vi "Streamlined FPGA--130415.vi"() -> ()   [LabVIEW 2009]
uses:
  Instance           2 24Saved   Streamlined FPGA .vi
  <vilib>/eio/EIONode/EIONode.xnode
  Instance           3 24Saved   Streamlined FPGA .vi
  Instance           4 24Saved   Streamlined FPGA .vi
  Instance           5 24Saved   Streamlined FPGA .vi
  <vilib>/rvi/eio/nirviEIOImplementation/nirviEIOImplementation.xnode
  <vilib>/rvi/eio/common/nirviEmuClasses.ctl
  <vilib>/rvi/eio/common/nirviEmuTemplateMethod_noerrors.vi
  <vilib>/rvi/DataTransferAndStorage/Container/XNode/niFpgaContainer.xnode
  <vilib>/rvi/DataTransferAndStorage/Container/Common/niFpgaTransferTypeControl.ctl
  <vilib>/rvi/DataTransferAndStorage/Container/Common/niFpgaContainerMethod.ctl
  <vilib>/rvi/interface/RandomDataEmulation/nirviRandomDataFPGAFIFO.vi
  <vilib>/rvi/interface/RandomDataEmulation/niFpgaRandomDataHandleErrors.vi
panel:
  in  "window size":i32
  in  "smooth":bool
  in  "Rec2 Ymin":i32
  in  "Rec2 Xmin":i32
  in  "Rec1 Ymin":i32
  in  "Rec1 Xmin":i32
  in  "Rec2 Ymax":i32
  in  "Rec1 Ymax":i32
  in  "Rec2 Xmax":i32
  in  "Rec1 Xmax":i32
  out "sort!":bool
  in  "Maximum Width":i16
  in  "Maximum Height":i16
  in  "trigger on all":bool
  out "sort pulse":i16
  in  "Baselines":i16[](array[numeric])=[0, 0, 0, 0]
  in  "Sb":i8(ring)=1 items=["PMT1", "PMT2", "PMT3", "PMT4"]
  in  "Sa":i8(ring) items=["PMT1", "PMT2", "PMT3", "PMT4"]
  in  "Sort Case":i8(ring)=1 items=["FP", "Magnitude"]
  out "Full 2":bool
  in  "sort?":bool
  out "Drop counter":u32
  out "sort counter":u32
  in  "PMT to detect drops on":u8
  in  "Minimum Height":i16
  in  "Minimum Width":i16
  in  "Ticks between acquires (Ticks)":u32=200
  in  "Gain 1":i16(slide) scale=-32767.0..32767.0
  in  "Gain 2":i16(slide) scale=-32767.0..32767.0
  in  "Gain 3":i16(slide) scale=-32767.0..32767.0
  in  "Gain 4":i16(slide) scale=-32767.0..32767.0
  in  "amplitude":i16
  in  "1/Frequency \n(ticks)":u32
  in  "Burst \nCycles":i32
  in  "delay [us]":u32=20 min=1 max=8000
  # "Acquisition and Detection"
  # "FP and Sorting Parameters"
  # "Sorting Pulse\nGenerator"
  # "Events"
  # "PMT Controls"
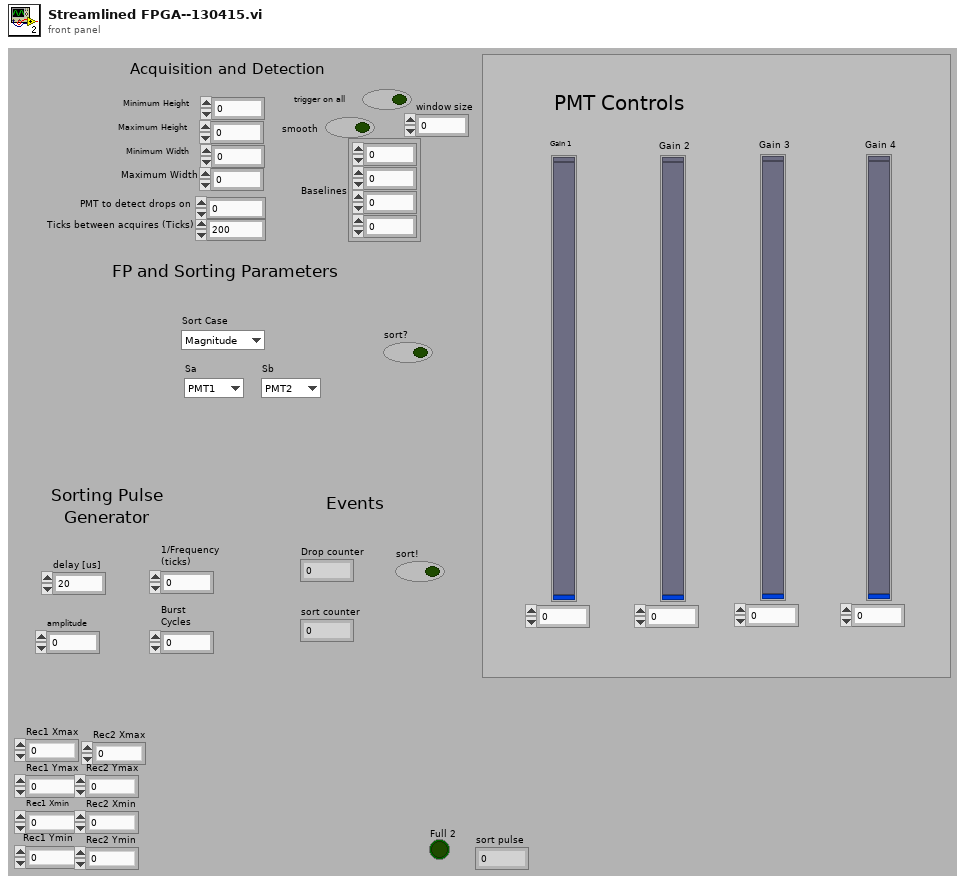
[diagram p1: front panel]
types:
  T1 = typedef "nirviEmuClasses.ctl" = enum16{"IO Read", "IO Write", "Method", "Property Read", "Property Write"}
  T2 = typedef "niFpgaContainerMethod.ctl" = enum16{"Write", "Read", "Clear", "Get Number of Elements to Write", "Get Number of Elements to Read", "Enable", "Disable", "Flush and Disable", "Get Stream State"}
  T3 = typedef "niFpgaTransferTypeControl.ctl" = enum16{"Target-Scoped", "Host to Target - DMA", "Target to Host - DMA", "Peer to Peer Reader", "Peer to Peer Writer", "Bidirectional"}
  T4 = cluster{"Rec1 Xmax":i32, "Rec1 Ymax":i32, "Rec1 Xmin":i32, "Rec1 Ymin":i32, "Rec2 Xmax":i32, "Rec2 Ymax":i32, "Rec2 Xmin":i32, "Rec2 Ymin":i32}
  T5 = cluster{bool, "max":i16[], "sum":i32[], "time inside":i32, "time outside":i32, "timeoutside-1":i32}
  T6 = cluster{"maxes":i16[], "sums":i32[], "time inside":i32, "time outside":i32}
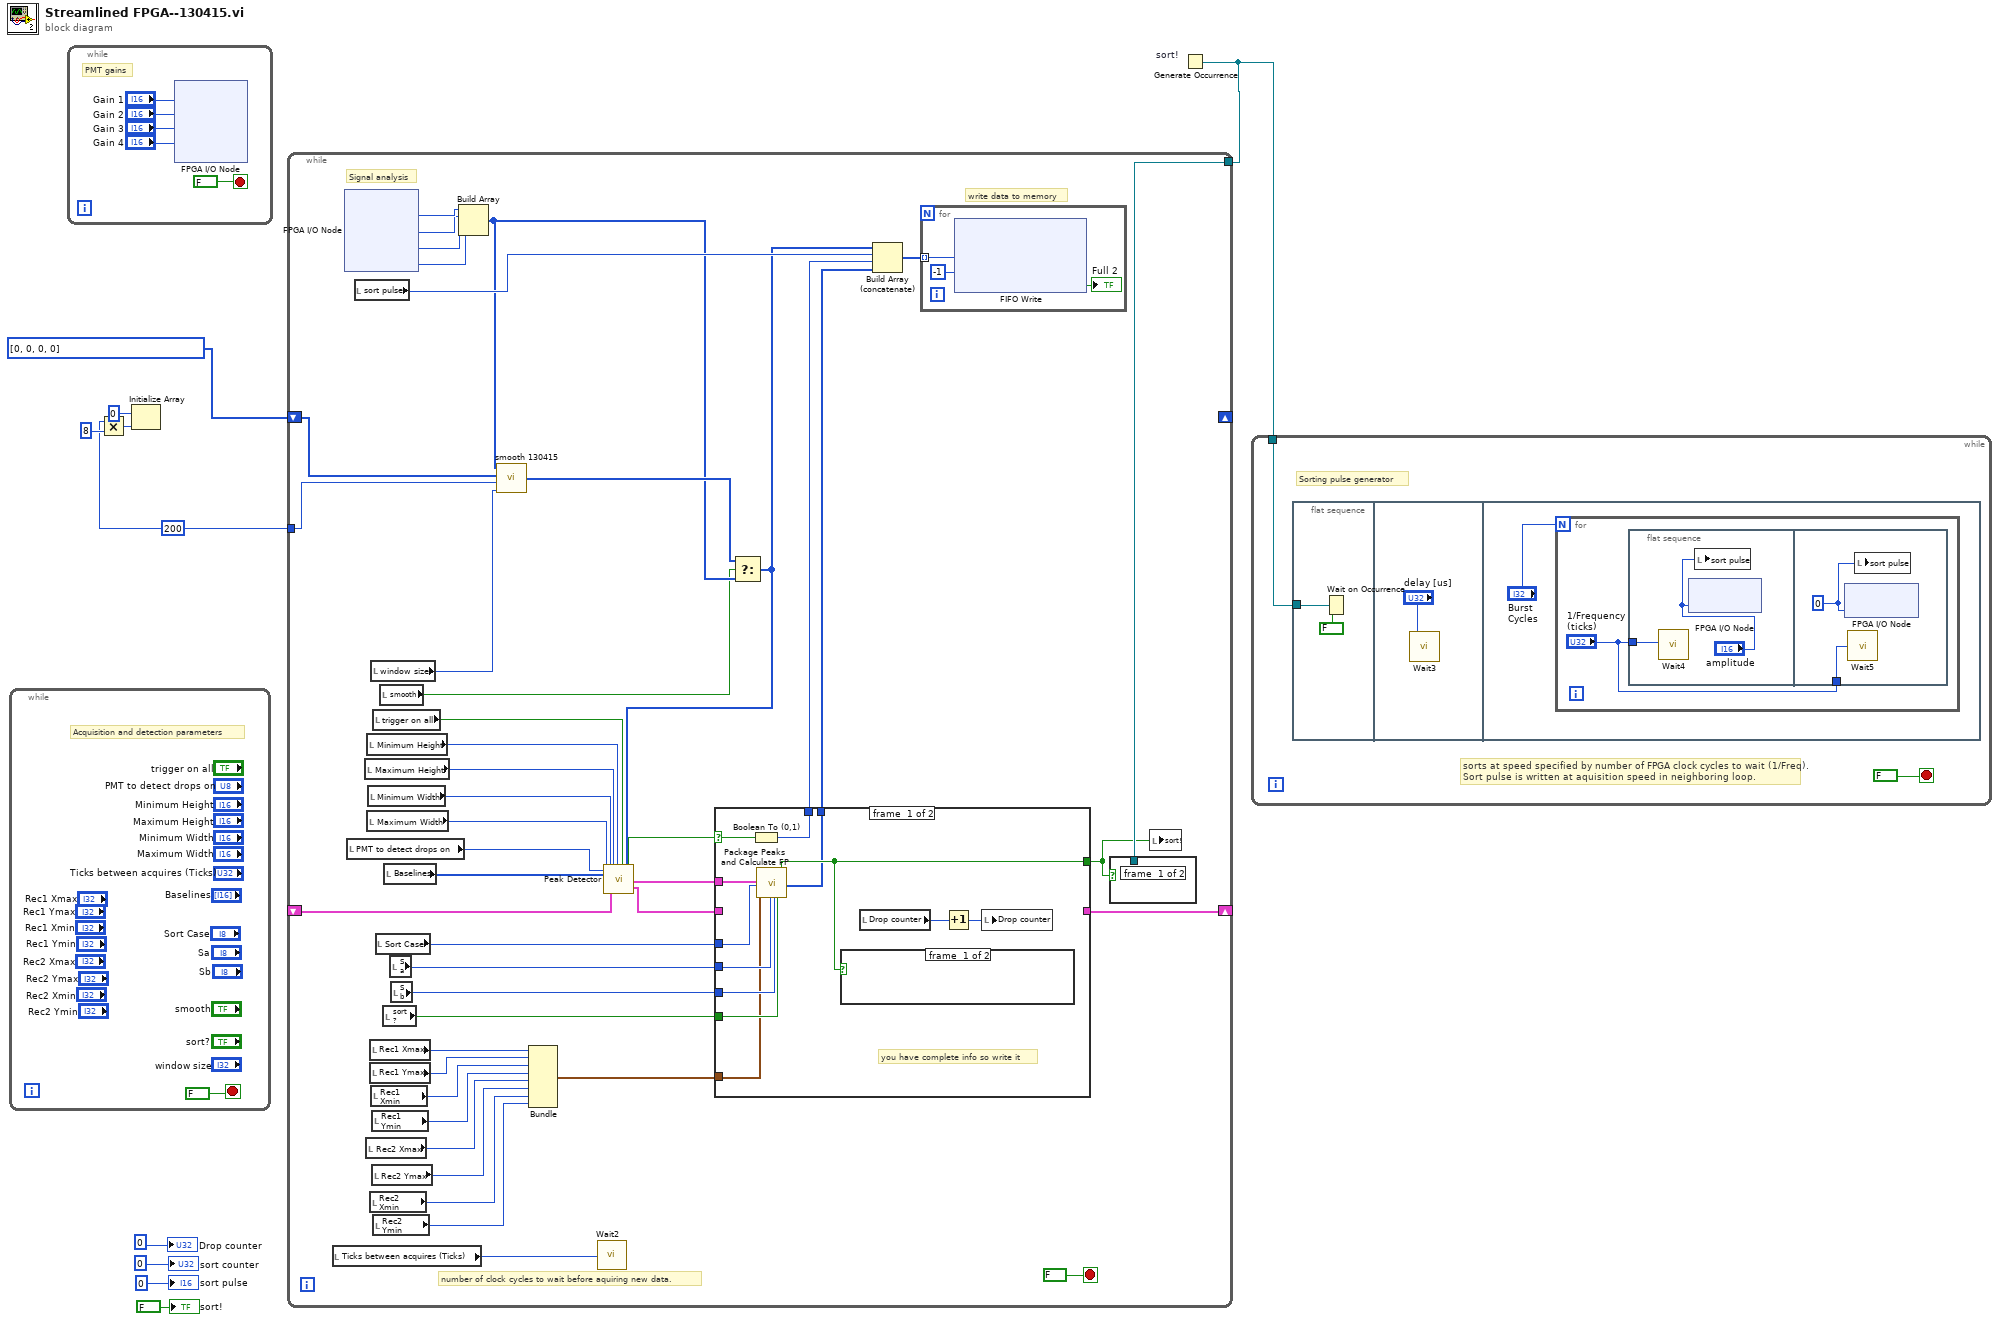
[diagram p0: block diagram]
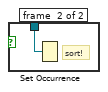
[diagram p2: hidden frame]
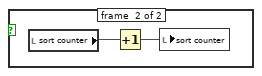
[diagram p3: hidden frame]
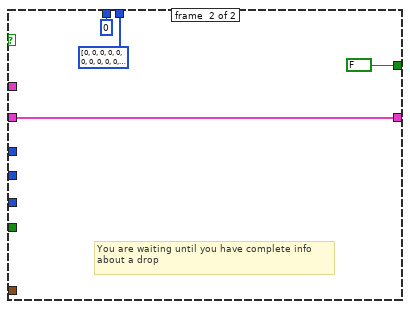
[diagram p4: hidden frame]
diagram:
  w2 = 200 ("dimension size")
  n1 = while {
    stop <- FALSE stop-if-true
    # "Acquisition and detection parameters"
  }
  n2 = while {
    stop <- FALSE stop-if-true
    # "PMT gains"
    n3 = xnode "FPGA I/O Node"("AO0"="Gain 1", "AO1"="Gain 2", "AO2"="Gain 3", "AO3"="Gain 4") -> ()  [unwired: 4 in, 4 out]
  }
  n4 = Multiply(x=w2, y=8 ("element")) -> (x*y=w3:i32)
  n5 = Initialize Array(0 ("element"), w3) -> ()  [unwired: 1 out]
  n6 = Generate Occurrence "sort!"() -> (w10:refnum<k4>)
  n7 = while {
    shift-right: [w103] -> _
    shift-left: _ -> [w90]
    tunnel: w10 -> [w88]
    shift-right: _ -> [_]
    shift-left: i32[] [0, 0, 0, 0] ("initialized array") -> [w67]
    tunnel: w2 -> [w66]
    stop <- FALSE stop-if-true
    # "number of clock cycles to wait before aquiring new data."
    # "Signal analysis"
    # "write data to memory"
    n8 = local read "Ticks between acquires (Ticks)"() -> (w98:u32)
    n9 = xnode "FPGA I/O Node"() -> ("AI0"=w102:i16, "AI1"=w101:i16, "AI2"=w100:i16, "AI3"=w99:i16)  [unwired: 4 in, 4 out]
    n10 = local read "PMT to detect drops on"() -> (w80:u8)
    n11 = local read "sort pulse"() -> (w87:i16)
    n12 = local read "Maximum Height"() -> (w83:i16)
    n13 = local read "Rec2 Xmax"() -> (w72:i32)
    n14 = local read "Minimum Height"() -> (w84:i16)
    n15 = local read "Maximum Width"() -> (w81:i16)
    n16 = local read "Minimum Width"() -> (w82:i16)
    n17 = local read "Rec1 Xmax"() -> (w76:i32)
    n18 = local read "Rec1 Ymax"() -> (w75:i32)
    n19 = local read "Rec2 Xmin"() -> (w70:i32)
    n20 = local read "window size"() -> (w65:i32)
    n21 = local read "Rec1 Xmin"() -> (w74:i32)
    n22 = local read "Rec1 Ymin"() -> (w73:i32)
    n23 = local read "Rec2 Ymax"() -> (w71:i32)
    n24 = local read "trigger on all"() -> (w89:bool)
    n25 = local read "Rec2 Ymin"() -> (w69:i32)
    n26 = local read "Sort Case"() -> (w97:i8)
    n27 = local read "smooth"() -> (w62:bool)
    n28 = local read "sort?"() -> (w94:bool)
    n29 = local read "Baselines"() -> (w79:i16[])
    n30 = local read "Sa"() -> (w96:i8)
    n31 = local read "Sb"() -> (w95:i8)
    n32 = Build Array(w102, w101, w100, w99) -> (w63:i16[])
    n33 = call "smooth 130415.vi"("window size"=w65, "dimension size"=w66, "initialized array"=w67, "Array"=w63) -> ("Array 2"=w64:i32[])
    n34 = Bundle("Rec1 Xmax"=w76, "Rec1 Ymax"=w75, "Rec1 Xmin"=w74, "Rec1 Ymin"=w73, "Rec2 Xmax"=w72, "Rec2 Ymax"=w71, "Rec2 Xmin"=w70, "Rec2 Ymin"=w69) -> (w68:T4)  [unwired: 1 in]
    n35 = call "Wait2"("Count(Ticks)"=w98) -> ()  [unwired: 1 out]
    n36 = Select(t=w64, s=w62, f=w63) -> (s? t:f=w61:i32[])
    n37 = call "Peak Detector.vi"("Maximum Width"=w81, "PMT to trigger on (0,1,2,3)"=w80, "Baselines"=w79, "Minimum Width"=w82, "shifts in"=w90, "Maximum Height"=w83, "Minimum Height"=w84, "trigger on all"=w89, "s1,s2,s3,s4"=w61) -> ("peak complete?"=w93:bool, "shifts out"=w91:T5, "peaks data"=w92:T6)  [unwired: 16 in]
    n38 = case shown="True" w93 {
      selector: w93 -> [w215 _]
      tunnel: [_ w226] -> w103
      tunnel: [w213 FALSE ("sort!")] -> w78
      tunnel: w97 -> [w211 _]
      tunnel: w96 -> [w219 _]
      tunnel: w95 -> [w218 _]
      tunnel: w94 -> [w217 _]
      tunnel: w91 -> [_ w226]
      tunnel: w92 -> [w216 _]
      tunnel: [w214 i16 0] -> w85
      tunnel: [w212 i32[] [0, 0, 0, 0, 0, 0, 0, 0, 0, 0, 0, 0] ("M1,M2,M3,M4,S1,S2,S3,S4,Tin,Tout,FP")] -> w77
      tunnel: w68 -> [w210 _]
      frame #0 {
        # "you have complete info so write it"
        n39 = Boolean To (0,1)(Boolean=w215) -> (0, 1=w214:i16)
        n40 = call "Package Peaks and Calculate FP.vi"("peaks data"=w216, "Sort Case"=w211, "Rectangle Positions"=w210, "Sa"=w219, "Sb"=w218, "sort?"=w217) -> ("sort!"=w213:bool, "M1,M2,M3,M4,S1,S2,S3,S4,Tin,Tout,FP,Sort?"=w212:i32[])  [unwired: 14 in, 6 out]
        n41 = case shown="True" w213 {
          frame #0 {
          }
          frame #1 {
            n42 = local read "sort counter"() -> (w223:u32)
            n43 = Increment(x=w223) -> (x+1=w222:u32)
            n44 = local write "sort counter"(w222) -> ()
          }
        }
        n45 = local read "Drop counter"() -> (w221:u32)
        n46 = Increment(x=w221) -> (x+1=w220:u32)
        n47 = local write "Drop counter"(w220) -> ()
      }
      frame #1 {
        # "You are waiting until you have complete info about a drop"
      }
    }
    n48 = Build Array (concatenate)(w61, w87, w85, w77) -> (w86:i32[])
    n49 = for {
      tunnel: w86 -> [w108] mode=indexing
      n50 = xnode ("FIFO Write")("Element"=w108, "Timeout"=-1) -> ("Timed Out?"=→"Full 2":bool)  [unwired: 1 in, 1 out]
    }
    n51 = case shown="True" w78 {
      tunnel: w88 -> [_ w105]
      frame #0 {
      }
      frame #1 {
        # "sort!"
        n52 = Set Occurrence(w105) -> ()
      }
    }
    n53 = local write "sort!"(w78) -> ()
  }
  n54 = while {
    tunnel: w10 -> [w228]
    stop <- FALSE stop-if-true
    # "sorts at speed specified by number of FPGA clock cycles to wait (1/Freq).\nSort pulse is written at aquisition speed in neighboring loop."
    # "Sorting pulse generator"
    n55 = flat-sequence {
      tunnel: w228 -> [w230]
      frame #0 {
        n56 = Wait on Occurrence(1:FALSE ("ignore previous (T)"), 2:w230) -> ()  [unwired: 1 in, 1 out]
      }
      frame #1 {
        n57 = call "Wait3"("Count(uSec)"="delay [us]") -> ()  [unwired: 1 out]
      }
      frame #2 {
        n58 = for {
          N: "Burst \nCycles" -> [_]
          n59 = flat-sequence {
            tunnel: "1/Frequency \n(ticks)" -> [w236]
            tunnel: "1/Frequency \n(ticks)" -> [w249]
            frame #0 {
              n60 = call "Wait4"("Count(Ticks)"=w236) -> ()  [unwired: 1 out]
              n61 = xnode "FPGA I/O Node"("AO4"="amplitude") -> ()  [unwired: 1 in, 1 out]
              n62 = local write "sort pulse"("amplitude") -> ()
            }
            frame #1 {
              w248 = i16 0 ("sort pulse")
              n63 = xnode "FPGA I/O Node"("AO4"=w248) -> ()  [unwired: 1 in, 1 out]
              n64 = call "Wait5"("Count(Ticks)"=w249) -> ()  [unwired: 1 out]
              n65 = local write "sort pulse"(w248) -> ()
            }
          }
        }
      }
    }
  }
  "sort counter" <- u32 0 ("event counter")
  "Drop counter" <- u32 0 ("Drop counter")
  "sort pulse" <- i16 0 ("event counter")
  "sort!" <- FALSE ("sort!")
